vi "Main.vi"() -> ()   [LabVIEW 2018, in "CAN FD.lvlib"]
uses:
  CAN FD.lvlib
  Typedef/CAN Data.ctl
  SubVI/RTsave Thread.vi
  SubVI/Save Buffer.vi
  SubVI/Clear Buffer.vi
  Setup Dialog.vi
  SubVI/zlgcan.lvlib
panel:
  in  "About":bool
  in  "Management":bool
  in  "Save":bool
  in  "Group":bool
  in  "Pause":bool
  in  "Clear":bool
  in  "RTsave":bool
  in  "Send":bool
  in  "Setup":bool
  in  "Format":i16(ring)=-1 caption="帧格式" items=["全部"=-1, "数据帧"=0, "远程帧"=1]
  in  "Type":i16(ring)=-1 caption="帧类型" items=["全部"=-1, "标准帧"=0, "扩展帧"=1]
  in  "Len":string
  in  "Direction":i16(ring)=-1 caption="CAN类型" items=["全部"=-1, "Tx"=0, "Rx"=1]
  in  "CANType":i16(ring)=-1 caption="CAN类型" items=["全部"=-1, "CAN"=0, "CANFD"=1, "CANFD加速"=2]
  in  "ID":string
  in  "Channel":string
  in  "Timestamp":string caption="时间标识"
  in  "Data":string
  in  "List":i32(listbox)
  in  "Scroll":i32(c297)
  # "列表过滤"
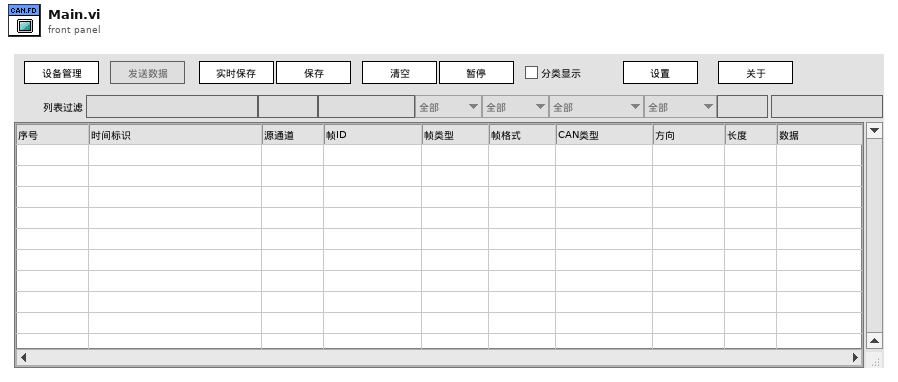
[diagram p1: front panel]
types:
  T1 = typedef "CAN FD.lvlib/CAN Data.ctl" = cluster{"SystemTime":timestamp, "HwTime":dbl, "Channel":u8, "ID":u32, "CANType":i16, "Direction":i16, "Remote":bool, "Ext":bool, "Len":u8, "Data":u8[], "Success":bool}
  T2 = enum32{"Invalid", "Standard", "Closed", "Hidden", "Minimized", "Maximized"}
  T3 = enum32{"Bad", "Idle", "Run top level", "Running"}
  T4 = typedef "CAN FD.lvlib/ListFilter.ctl" = cluster{"Timestamp":string, "Channel":string, "ID":string, "Type":i16, "Format":i16, "CANType":i16, "Direction":i16, "Len":string, "Data":string}
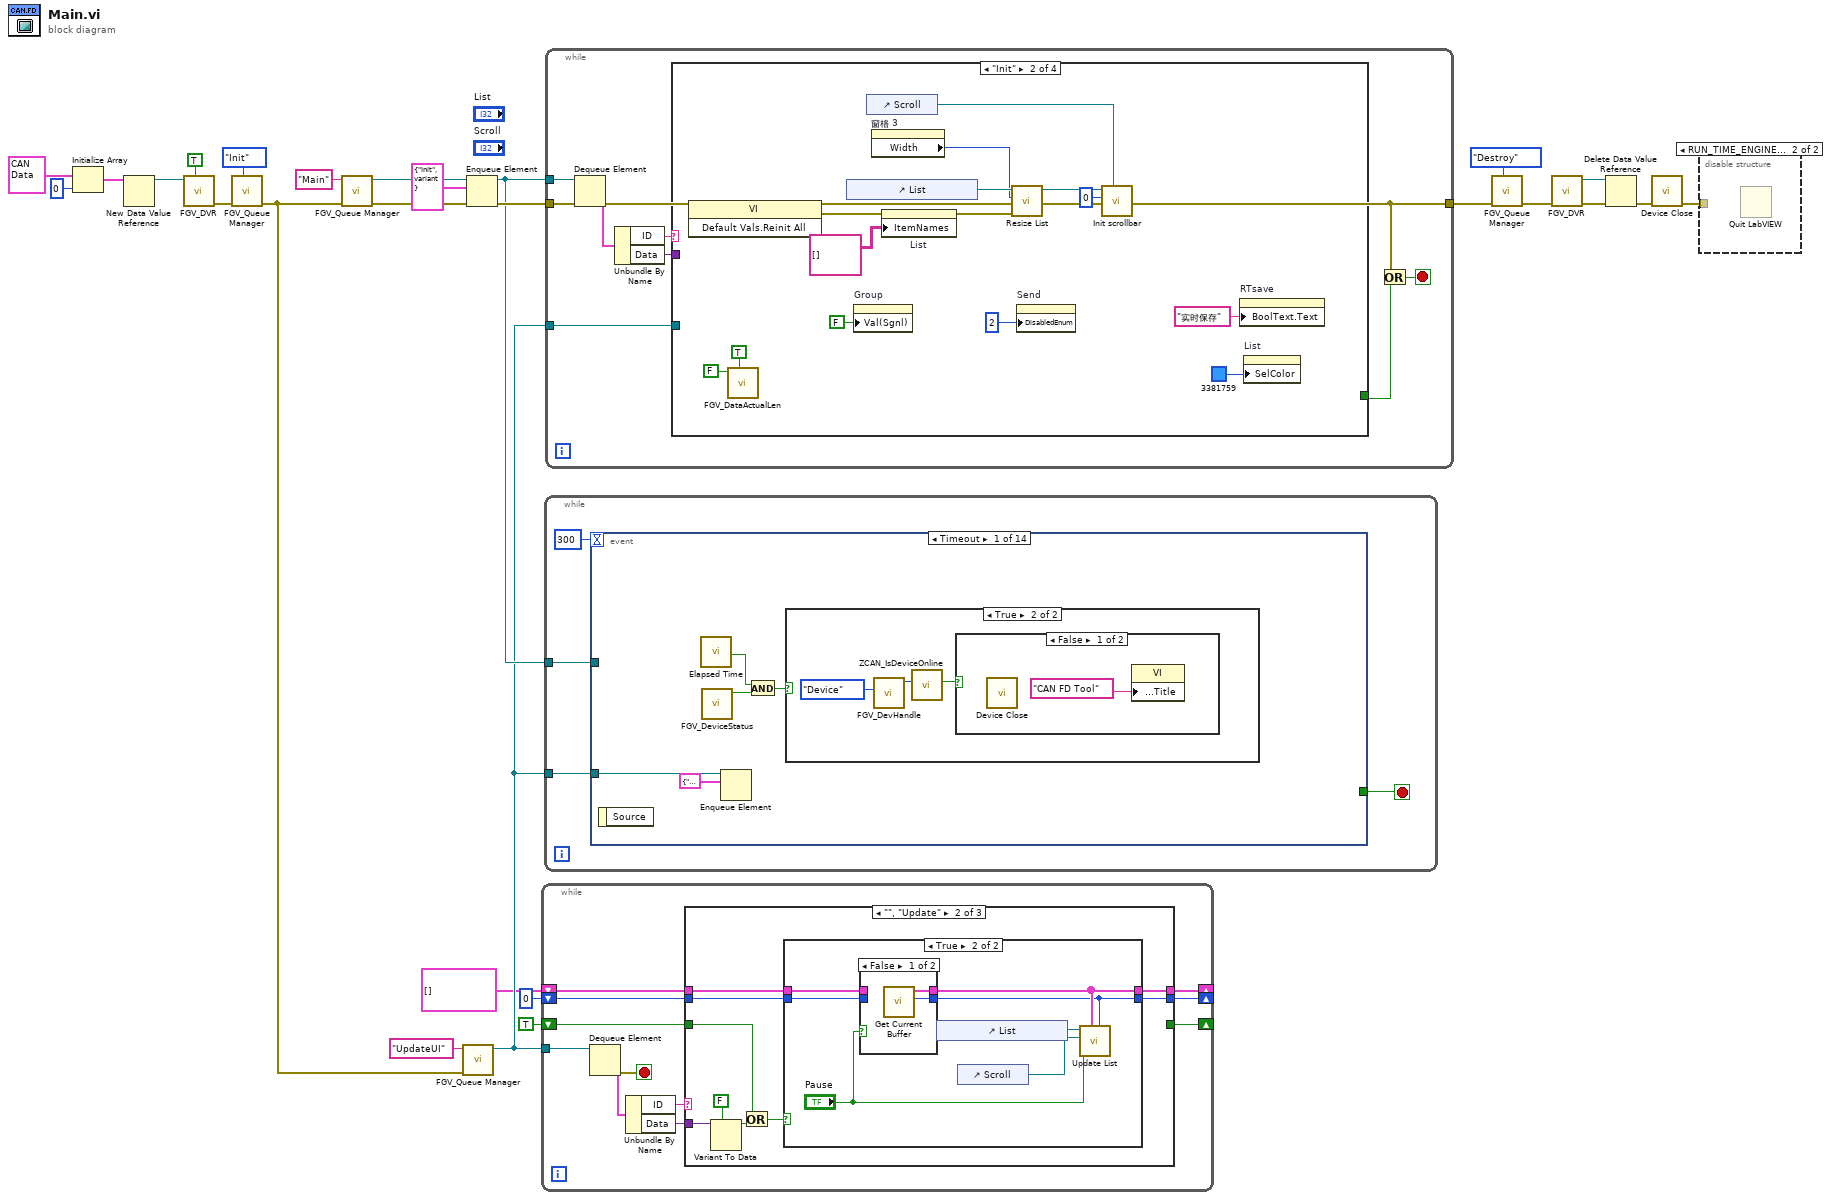
[diagram p0: block diagram]
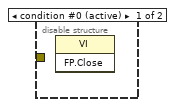
[diagram p2: hidden frame]
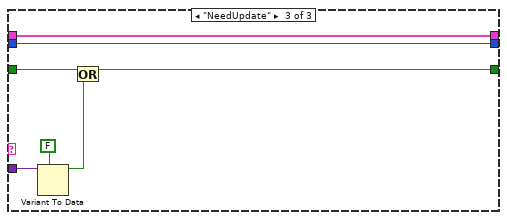
[diagram p6: hidden frame]
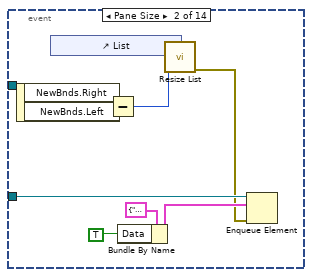
[diagram p9: hidden frame]
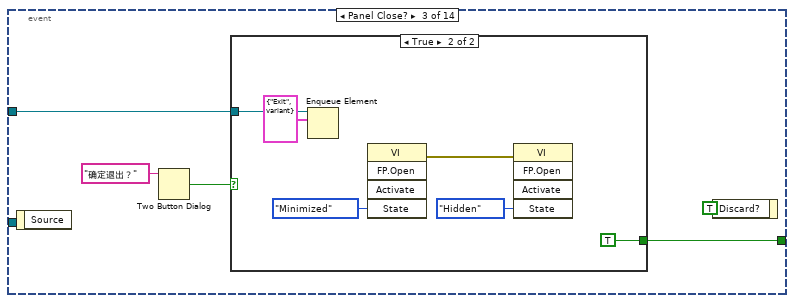
[diagram p10: hidden frame]
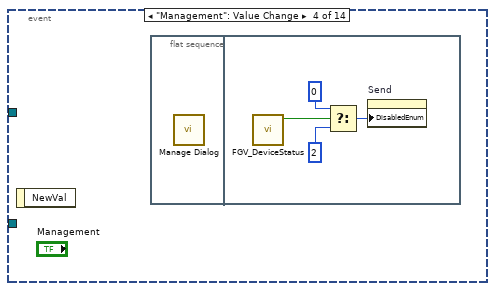
[diagram p12: hidden frame]
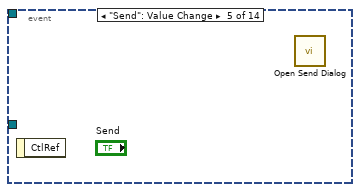
[diagram p13: hidden frame]
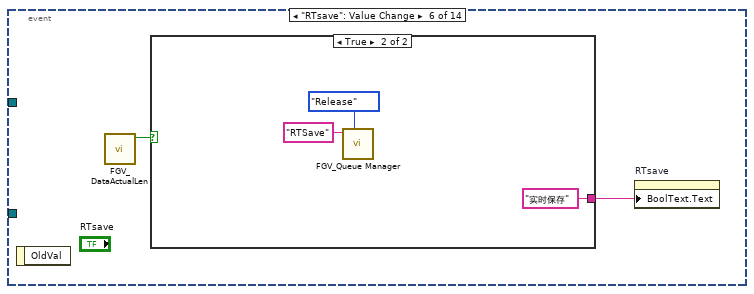
[diagram p14: hidden frame]
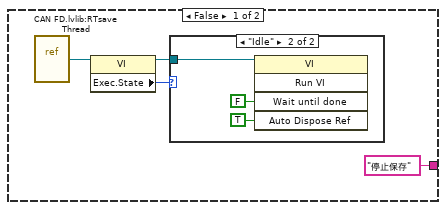
[diagram p15: hidden frame]
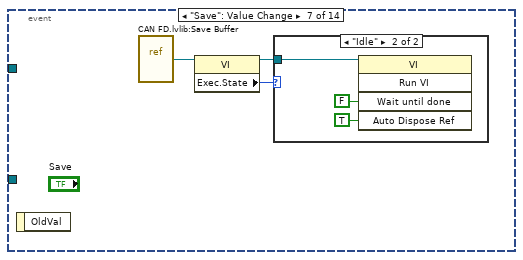
[diagram p17: hidden frame]
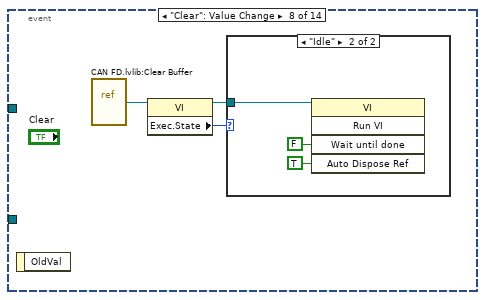
[diagram p19: hidden frame]
diagram:
  n1 = Initialize Array(T1 {"SystemTime"=timestamp(0 s since 1904-01-01), "HwTime"=0.0, "Channel"=0, "ID"=0, "CANType"=0, "Direction"=0, "Remote"=FALSE, "Ext"=FALSE, "Len"=0, "Data"=[], "Success"=FALSE} ("Data"), 0 ("维数大小")) -> (w17:T1[])
  n2 = New Data Value Reference(data value=w17) -> (data value reference=w16:refnum<data-value>)  [unwired: 1 in, 1 out]
  n3 = call "FGV_DVR.vi"("Set"=TRUE, "DVR"=w16) -> ("error out"=w15:errorcluster)  [unwired: 8 in, 1 out]
  n4 = call "FGV_Queue Manager.vi"("Methods"=enum16{"Init", "Get", "Release", "Destroy"}."Init", "error in (no error)"=w15) -> ("error out"=w9:errorcluster)  [unwired: 7 in, 2 out]
  n5 = call "FGV_Queue Manager.vi"("error in (no error)"=w9, "Name"="Main") -> ("error out"=w24:errorcluster, "Queue"=w25:refnum<queue>)  [unwired: 7 in, 1 out]
  n6 = call "FGV_Queue Manager.vi"("error in (no error)"=w9, "Name"="UpdateUI") -> ("Queue"=w8:refnum<queue>)  [unwired: 7 in, 2 out]
  n7 = Enqueue Element(queue=w25, element=cluster{"ID":string, "Data":variant} {"ID"="Init", "Data"=variant} ("元素"), error in (no error)=w24) -> (queue out=w20:refnum<queue>, error out=w22:errorcluster)  [unwired: 1 in, 1 out]
  n8 = while {
    tunnel: w8 -> [w37]
    shift-right: [w31] -> _
    shift-left: TRUE -> [w32]
    shift-right: [w30] -> _
    shift-left: T1[] [] ("Data") -> [w29]
    shift-right: [w28] -> _
    shift-left: 0 ("ZeroOffset") -> [w27]
    stop <- w34 stop-if-true
    n9 = Dequeue Element(queue=w37) -> (element=w36:cluster{"ID":string, "Data":variant}, error out=w34:errorcluster)  [unwired: 2 in, 2 out]
    n10 = Unbundle By Name(w36) -> ("ID"=w35:string, "Data"=w33:variant)
    n11 = case shown="\"\", \"Update\"" w35 {
      tunnel: w33 -> [_ w48 w69]
      tunnel: w32 -> [w40 w46 w67]
      tunnel: [w40 _ w65] -> w31
      tunnel: [w39 w44 w64] -> w30
      tunnel: w29 -> [w39 w43 w64]
      tunnel: [w38 w42 w63] -> w28
      tunnel: w27 -> [w38 w41 w63]
      frame Default {
      }
      frame "", "Update" {
        n12 = Variant To Data(type=FALSE, Variant=w48) -> (data=w47:bool)  [unwired: 1 in, 1 out]
        n13 = Or(x=w46, y=w47) -> (x .or. y?=w45:bool)
        n14 = case shown="True" w45 {
          tunnel: [w51 w55] -> w44
          tunnel: w43 -> [w51 w56]
          tunnel: [w50 w53] -> w42
          tunnel: w41 -> [w50 w54]
          frame False {
          }
          frame True {
            n15 = case shown="False" "Pause" {
              tunnel: [w60 w62] -> w55
              tunnel: w56 -> [_ w62]
              tunnel: [w59 w61] -> w53
              tunnel: w54 -> [_ w61]
              frame False {
                n16 = call "Get Current Buffer.vi"() -> ("ZeroOffset"=w59:i32, "Data"=w60:T1[])  [unwired: 10 in]
              }
              frame True {
              }
            }
            n17 = control-ref of="List"() -> (w57:refnum<vi>)
            n18 = control-ref of="Scroll"() -> (w58:refnum<vi>)
            n19 = call "Update List.vi"("ZeroOffset"=w53, "Data"=w55, "Pause"="Pause", "Scroll"=w58, "List"=w57) -> ()  [unwired: 7 in]
          }
        }
      }
      frame "NeedUpdate" {
        n20 = Variant To Data(type=FALSE, Variant=w69) -> (data=w66:bool)  [unwired: 1 in, 1 out]
        n21 = Or(x=w67, y=w66) -> (x .or. y?=w65:bool)
      }
    }
  }
  n22 = while {
    tunnel: w20 -> [w73]
    tunnel: w8 -> [w71]
    stop <- w72 stop-if-true
    n23 = event shown="[0] Timeout" {
      selector: _ -> [_ _ _ _ _ _ _ _ _ _ _ _ _ _]
      dyn-events: _ -> [_ _ _ _ _ _ _ _ _ _ _ _ _ _]
      timeout: 300 -> [_ _ _ _ _ _ _ _ _ _ _ _ _ _]
      tunnel: w73 -> [_ _ w94 _ _ _ _ _ _ _ _ _ _ _]
      tunnel: [_ _ w93 _ _ _ _ _ _ _ _ _ _ _] -> w72
      tunnel: w71 -> [w77 w84 _ _ _ _ _ _ w131 _ w162 w166 w171 _]
      event Timeout {
        n24 = event-data() -> ()  [unwired: 1 in, 1 out]
        n25 = call "Elapsed Time"() -> ("Time has Elapsed"=w76:bool)  [unwired: 12 in, 7 out]
        n26 = call "FGV_DeviceStatus.vi"() -> ("Open?"=w75:bool)  [unwired: 10 in, 1 out]
        n27 = Enqueue Element(queue=w77, element=cluster{"ID":string, "Data":variant} {"ID"="Update", "Data"=variant} ("元素")) -> ()  [unwired: 2 in, 3 out]
        n28 = And(x=w76, y=w75) -> (x .and. y?=w74:bool)
        n29 = case shown="True" w74 {
          frame False {
          }
          frame True {
            n30 = call "FGV_DevHandle.vi"("Type"=enum16{"Device", "Ch0", "Ch1"}."Device") -> ("handle out"=w80:u64)  [unwired: 8 in, 2 out]
            n31 = call "ZCAN_IsDeviceOnline.vi"("device_handle"=w80) -> ("Online?"=w79:bool)  [unwired: 9 in, 1 out]
            n32 = case shown="False" w79 {
              frame False {
                n33 = call "Device Close.vi"() -> ()  [unwired: 11 in, 1 out]
                n34 = property class="VI"("Front Panel.Title"="CAN FD Tool") -> ()  [unwired: 2 in, 2 out]
              }
              frame True {
              }
            }
          }
        }
      }
      event Pane Size {
        n35 = event-data() -> ("NewBnds.Right"=w89:i16, "NewBnds.Left"=w90:i16)  [unwired: 1 in]
        n36 = control-ref of="List"() -> (w91:refnum<vi>)
        n37 = Subtract(x=w89, y=w90) -> (x-y=w88:i16)
        n38 = Bundle By Name(cluster=cluster{"ID":string, "Data":variant} {"ID"="Update", "Data"=variant} ("元素"), "Data"=TRUE) -> (w85:cluster{"ID":string, "Data":variant})
        n39 = call "Resize List.vi"("Panel Width"=w88, "List"=w91) -> ("error out"=w83:errorcluster)  [unwired: 8 in, 1 out]
        n40 = Enqueue Element(queue=w84, element=w85, error in (no error)=w83) -> ()  [unwired: 1 in, 3 out]
      }
      event Panel Close? {
        n41 = event-data() -> ()  [unwired: 1 in, 1 out]
        n42 = Two Button Dialog(message="确定退出？" ("消息")) -> (T button?=w95:bool)  [unwired: 2 in]
        n43 = case shown="True" w95 {
          tunnel: w94 -> [_ w102]
          tunnel: [_ TRUE] -> w93
          frame False {
          }
          frame True {
            n44 = Enqueue Element(queue=w102, element=cluster{"ID":string, "Data":variant} {"ID"="Exit", "Data"=variant} ("元素")) -> ()  [unwired: 2 in, 3 out]
            n45 = invoke class="VI" method="FP.Open"("State"=T2."Minimized" ("州")) -> (error out=w98:errorcluster)  [unwired: 4 in, 4 out]
            n46 = invoke class="VI" method="FP.Open"(error in=w98, "State"=T2."Hidden" ("州")) -> ()  [unwired: 3 in, 5 out]
          }
        }
        n47 = event-data("Discard?"=TRUE ("放弃？")) -> ()  [unwired: 1 in, 1 out]
      }
      event "Management": Value Change {
        n48 = event-data() -> ()  [unwired: 1 in, 1 out]
        n49 = flat-sequence {
          frame #0 {
            n50 = call "Manage Dialog.vi"() -> ()  [unwired: 12 in]
          }
          frame #1 {
            n51 = call "FGV_DeviceStatus.vi"() -> ("Open?"=w104:bool)  [unwired: 10 in, 1 out]
            n52 = Select(t=0, s=w104, f=2) -> (s? t:f=w103:i32)
            n53 = property on="Send" class="Bool"("DisabledEnum"=w103) -> ()  [unwired: 2 in, 2 out]
          }
        }
      }
      event "Send": Value Change {
        n54 = event-data() -> ()  [unwired: 1 in, 1 out]
        n55 = call "Open Send Dialog.vi"() -> ()  [unwired: 12 in]
      }
      event "RTsave": Value Change {
        n56 = event-data() -> ()  [unwired: 1 in, 1 out]
        n57 = call "FGV_DataActualLen.vi"() -> ("RTsave"=w108:bool)  [unwired: 10 in, 1 out]
        n58 = case shown="True" w108 {
          tunnel: ["停止保存" ("布尔文本.文本") "实时保存" ("布尔文本.文本")] -> w107
          frame False {
            n59 = vi-ref "CAN FD.lvlib:RTsave Thread.vi"() -> (w111:refnum<vi>)
            n60 = property class="VI"(reference=w111) -> (reference out=w109:refnum<vi>, "Exec.State"=w110:T3)  [unwired: 1 in, 1 out]
            n61 = case shown="\"Idle\"" w110 {
              tunnel: w109 -> [_ w115]
              frame "Bad", Default {
              }
              frame "Idle" {
                n62 = invoke class="VI" method="Run VI"(reference=w115, "Wait until done"=FALSE ("结束前等待"), "Auto Dispose Ref"=TRUE ("自动销毁引用")) -> ()  [unwired: 2 in, 5 out]
              }
            }
          }
          frame True {
            n63 = call "FGV_Queue Manager.vi"("Methods"=enum16{"Init", "Get", "Release", "Destroy"}."Release", "Name"="RTSave") -> ()  [unwired: 7 in, 3 out]
          }
        }
        n64 = property on="RTsave" class="Bool"("BoolText.Text"=w107) -> ()  [unwired: 2 in, 2 out]
      }
      event "Save": Value Change {
        n65 = event-data() -> ()  [unwired: 1 in, 1 out]
        n66 = vi-ref "CAN FD.lvlib:Save Buffer.vi"() -> (w121:refnum<vi>)
        n67 = property class="VI"(reference=w121) -> (reference out=w119:refnum<vi>, "Exec.State"=w120:T3)  [unwired: 1 in, 1 out]
        n68 = case shown="\"Idle\"" w120 {
          tunnel: w119 -> [_ w124]
          frame "Bad", Default {
          }
          frame "Idle" {
            n69 = invoke class="VI" method="Run VI"(reference=w124, "Wait until done"=FALSE ("结束前等待"), "Auto Dispose Ref"=TRUE ("自动销毁引用")) -> ()  [unwired: 2 in, 5 out]
          }
        }
      }
      event "Clear": Value Change {
        n70 = event-data() -> ()  [unwired: 1 in, 1 out]
        n71 = vi-ref "CAN FD.lvlib:Clear Buffer.vi"() -> (w127:refnum<vi>)
        n72 = property class="VI"(reference=w127) -> (reference out=w125:refnum<vi>, "Exec.State"=w126:T3)  [unwired: 1 in, 1 out]
        n73 = case shown="\"Idle\"" w126 {
          tunnel: w125 -> [_ w130]
          frame "Bad", Default {
          }
          frame "Idle" {
            n74 = invoke class="VI" method="Run VI"(reference=w130, "Wait until done"=FALSE ("结束前等待"), "Auto Dispose Ref"=TRUE ("自动销毁引用")) -> ()  [unwired: 2 in, 5 out]
          }
        }
      }
      event "Group": Value Change {
        n75 = event-data() -> ("NewVal"=w140:bool)  [unwired: 1 in]
        n76 = call "FGV_Group Show.vi"("Set"=TRUE, "Group Show"=w140) -> ("Group Show"=w138:bool)  [unwired: 8 in, 1 out]
        n77 = Bundle By Name(cluster=cluster{"ID":string, "Data":variant} {"ID"="Update", "Data"=variant} ("元素"), "Data"=TRUE) -> (w132:cluster{"ID":string, "Data":variant})
        n78 = Enqueue Element(queue=w131, element=w132) -> ()  [unwired: 2 in, 3 out]
        n79 = Select(t=0, s=w138, f=2) -> (s? t:f=w135:i32)
        n80 = property on="Timestamp" class="Str"("DisabledEnum"=w135) -> ()  [unwired: 2 in, 2 out]
        n81 = property on="Channel" class="Str"("DisabledEnum"=w135) -> ()  [unwired: 2 in, 2 out]
        n82 = property on="ID" class="Str"("DisabledEnum"=w135) -> ()  [unwired: 2 in, 2 out]
        n83 = property on="CANType" class="Ring (strict)"("DisabledEnum"=w135) -> ()  [unwired: 2 in, 2 out]
        n84 = property on="Direction" class="Ring (strict)"("DisabledEnum"=w135) -> ()  [unwired: 2 in, 2 out]
        n85 = property on="Len" class="Str"("DisabledEnum"=w135) -> ()  [unwired: 2 in, 2 out]
        n86 = property on="Data" class="Str"("DisabledEnum"=w135) -> ()  [unwired: 2 in, 2 out]
        n87 = property on="Type" class="Ring (strict)"("DisabledEnum"=w135) -> ()  [unwired: 2 in, 2 out]
        n88 = property on="Format" class="Ring (strict)"("DisabledEnum"=w135) -> ()  [unwired: 2 in, 2 out]
      }
      event "Setup": Value Change {
        n89 = event-data() -> ()  [unwired: 1 in, 1 out]
        n90 = vi-ref "CAN FD.lvlib:Setup Dialog.vi"() -> (w143:refnum<vi>)
        n91 = property class="VI"(reference=w143) -> (reference out=w141:refnum<vi>, "Exec.State"=w142:T3)  [unwired: 1 in, 1 out]
        n92 = case shown="\"Idle\"" w142 {
          tunnel: w141 -> [_ w146]
          frame "Bad", Default {
          }
          frame "Idle" {
            n93 = invoke class="VI" method="Run VI"(reference=w146, "Wait until done"=FALSE ("结束前等待"), "Auto Dispose Ref"=TRUE ("自动销毁引用")) -> ()  [unwired: 2 in, 5 out]
          }
        }
      }
      event "Timestamp", "Channel", "ID", "CANType", "Direction", "Len", "Data", "Type", "Format": Value Change {
        n94 = event-data() -> ()  [unwired: 1 in, 1 out]
        n95 = call "FGV_ListFilter.vi"() -> ("Filter out"=w148:T4)  [unwired: 10 in, 1 out]
        n96 = Bundle(cluster=w148, "Timestamp"="Timestamp", "Channel"="Channel", "ID"="ID", "Type"="Type", "Format"="Format", "CANType"="CANType", "Direction"="Direction", "Len"="Len", "Data"="Data") -> (w147:T4)
        n97 = Bundle By Name(cluster=cluster{"ID":string, "Data":variant} {"ID"="Update", "Data"=variant} ("元素"), "Data"=TRUE) -> (w159:cluster{"ID":string, "Data":variant})
        n98 = call "FGV_ListFilter.vi"("Set"=TRUE, "Filter"=w147) -> ("error out"=w158:errorcluster)  [unwired: 8 in, 1 out]
        n99 = Enqueue Element(queue=w162, element=w159, error in (no error)=w158) -> ()  [unwired: 1 in, 3 out]
      }
      event "Scroll": Value Change {
        n100 = event-data() -> ()  [unwired: 1 in, 1 out]
        n101 = Bundle By Name(cluster=cluster{"ID":string, "Data":variant} {"ID"="Update", "Data"=variant} ("元素"), "Data"=TRUE) -> (w167:cluster{"ID":string, "Data":variant})
        n102 = Get Date/Time In Seconds() -> (seconds since 1Jan1904=w164:timestamp)
        n103 = Enqueue Element(queue=w166, element=w167) -> ()  [unwired: 2 in, 3 out]
        n104 = call "FGV_OperateTime.vi"("Set"=TRUE, "OperateTime"=w164) -> ()  [unwired: 8 in, 2 out]
      }
      event "Pause": Value Change {
        n105 = event-data() -> ("NewVal"=w170:bool)  [unwired: 1 in]
        n106 = case shown="False" w170 {
          tunnel: w171 -> [w172 _]
          frame False {
            n107 = Bundle By Name(cluster=cluster{"ID":string, "Data":variant} {"ID"="Update", "Data"=variant} ("元素"), "Data"=TRUE) -> (w173:cluster{"ID":string, "Data":variant})
            n108 = Enqueue Element(queue=w172, element=w173) -> ()  [unwired: 2 in, 3 out]
          }
          frame True {
          }
        }
      }
      event "About": Value Change {
        n109 = event-data() -> ()  [unwired: 1 in, 1 out]
        n110 = call "About.vi"() -> ()  [unwired: 12 in]
      }
    }
  }
  n111 = while {
    tunnel: w20 -> [w183]
    tunnel: w22 -> [w184]
    tunnel: [w179] -> w21
    tunnel: w8 -> [w176]
    stop <- w177 stop-if-true
    n112 = Dequeue Element(queue=w183, error in (no error)=w184) -> (element=w182:cluster{"ID":string, "Data":variant}, error out=w179:errorcluster)  [unwired: 1 in, 2 out]
    n113 = Unbundle By Name(w182) -> ("ID"=w181:string, "Data"=w180:variant)
    n114 = case shown="\"Init\"" w181 {
      tunnel: w180 -> [_ _ w207 _]
      tunnel: [_ _ _ TRUE] -> w178
      tunnel: w176 -> [_ _ w204 _]
      frame Default {
      }
      frame "Init" {
        n115 = invoke class="VI" method="Default Vals.Reinit All"() -> (error out=w198:errorcluster)  [unwired: 3 in, 2 out]
        n116 = call "FGV_DataActualLen.vi"("Set"=TRUE, "RTsave"=FALSE) -> ()  [unwired: 8 in, 2 out]
        n117 = control-ref of="List"() -> (w196:refnum<vi>)
        n118 = property on="Group" class="Bool (strict)"("Val(Sgnl)"=FALSE ("值(信号)")) -> ()  [unwired: 2 in, 2 out]
        n119 = control-ref of="Scroll"() -> (w192:refnum<vi>)
        n120 = property on="窗格 3" class="Pane"() -> ("Width"=w194:u32)  [unwired: 2 in, 2 out]
        n121 = property on="List" class="MCListbox (strict)"(error in=w198, "ItemNames"=string[][] [] ("项名")) -> (error out=w195:errorcluster)  [unwired: 1 in, 1 out]
        n122 = call "Resize List.vi"("error in (no error)"=w195, "Panel Width"=w194, "List"=w196) -> ("List out"=w193:refnum<vi>)  [unwired: 7 in, 1 out]
        n123 = property on="Send" class="Bool"("DisabledEnum"=2) -> ()  [unwired: 2 in, 2 out]
        n124 = call "Init scrollbar.vi"("Scroll"=w192, "Data Len"=0, "List"=w193) -> ()  [unwired: 7 in, 2 out]
        n125 = property on="RTsave" class="Bool"("BoolText.Text"="实时保存" ("布尔文本.文本")) -> ()  [unwired: 2 in, 2 out]
        n126 = property on="List" class="MCListbox (strict)"("SelColor"=u32 3381759) -> ()  [unwired: 2 in, 2 out]
      }
      frame "Data" {
        n127 = Variant To Data(type=T1[] [], Variant=w207) -> (data=w199:T1[], error out=w205:errorcluster)  [unwired: 1 in]
        n128 = call "New Data arrived.vi"("error in (no error)"=w205, "Data"=w199) -> ("error out"=w203:errorcluster)  [unwired: 9 in]
        n129 = Bundle By Name(cluster=cluster{"ID":string, "Data":variant} {"ID"="NeedUpdate", "Data"=variant} ("元素"), "Data"=TRUE) -> (w200:cluster{"ID":string, "Data":variant})
        n130 = Enqueue Element(queue=w204, element=w200, error in (no error)=w203) -> ()  [unwired: 1 in, 3 out]
      }
      frame "Exit", "Stop" {
      }
    }
    n131 = Or(x=w179, y=w178) -> (x .or. y?=w177:bool)
  }
  n132 = call "FGV_Queue Manager.vi"("Methods"=enum16{"Init", "Get", "Release", "Destroy"}."Destroy", "error in (no error)"=w21) -> ("error out"=w13:errorcluster)  [unwired: 7 in, 2 out]
  n133 = call "FGV_DVR.vi"("error in (no error)"=w13) -> ("error out"=w12:errorcluster, "DVR"=w11:refnum<data-value>)  [unwired: 9 in]
  n134 = Delete Data Value Reference(data value reference=w11, error in=w12) -> (error out=w3:errorcluster)  [unwired: 1 out]
  n135 = call "Device Close.vi"("error in (no error)"=w3) -> ("error out"=w2:errorcluster)  [unwired: 10 in]
  n136 = disable-structure shown="RUN_TIME_ENGINE==True" {
    disable-tunnel: w2 -> [_ _]
    frame condition #0 (active) {
      n137 = invoke class="VI" method="FP.Close"() -> ()  [unwired: 3 in, 3 out]
    }
    frame condition #1 {
      n138 = Quit LabVIEW() -> ()  [unwired: 1 in]
    }
  }
